vi "5_2.vi"() -> ()   [LabVIEW 2018]
uses:
  <vilib>/ptbypt/NI_PtbyPt.lvlib
  <vilib>/gmath/NI_Gmath.lvlib
panel:
  out "理论误码率":dbl
  out "噪声标准差":dbl
  out "理论门限误码率（设计误码率）":dbl
  out "理论最优门限":dbl
  out "先验概率P(H1)":dbl
  in  "先验概率P(H0)":dbl=0.5
  in  "噪声方差":dbl=0.02
  in  "样本数":u64=1000000
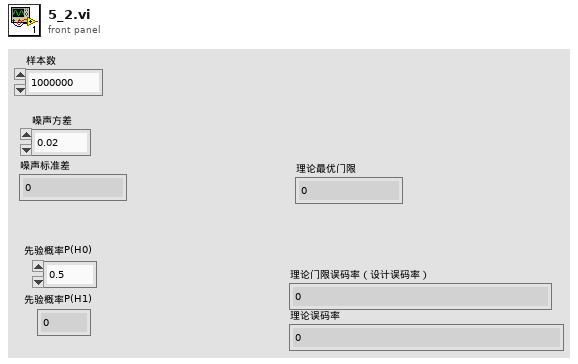
[diagram p1: front panel]
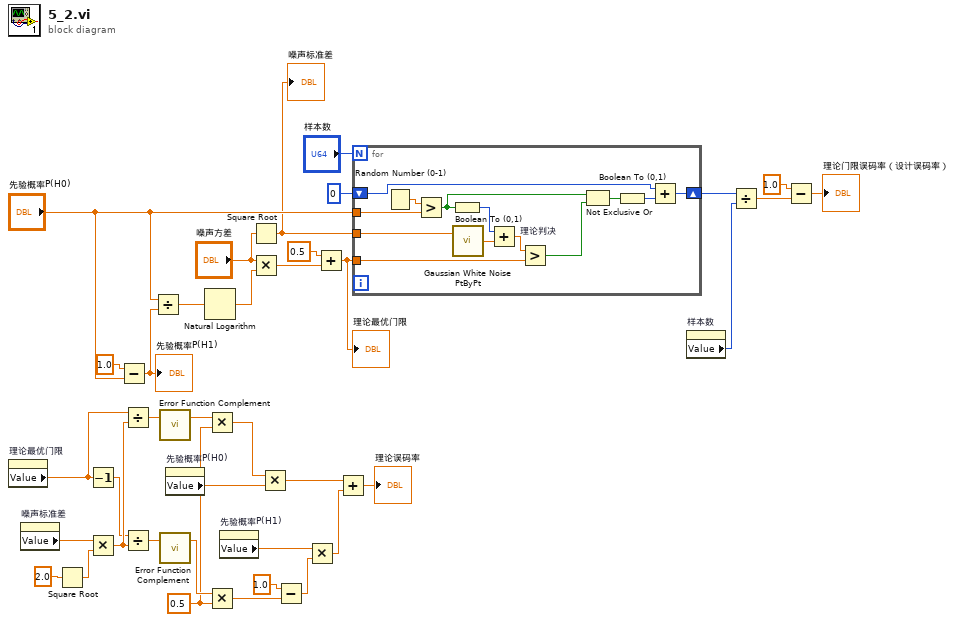
[diagram p0: block diagram]
diagram:
  w13 = 0.5 ("y")
  n1 = property on="理论最优门限" class="DigNum (严格)"() -> ("Value"=w19:dbl)  [unwired: 2 in, 2 out]
  n2 = property on="噪声标准差" class="DigNum (严格)"() -> ("Value"=w22:dbl)  [unwired: 2 in, 2 out]
  n3 = Square Root(x=2.0) -> (sqrt(x)=w21:dbl)
  n4 = Decrement(x=w19) -> (x-1=w18:dbl)
  n5 = Multiply(x=w22, y=w21) -> (x*y=w20:dbl)
  n6 = Subtract(x=1.0, y="先验概率P(H0)") -> (x-y=w29:dbl)
  "先验概率P(H1)" <- w29
  n7 = Divide(x=w19, y=w20) -> (x/y=w17:dbl)
  n8 = Divide(x=w18, y=w20) -> (x/y=w16:dbl)
  n9 = Divide(x="先验概率P(H0)", y=w29) -> (x/y=w35:dbl)
  n10 = call <vilib>:"Error Function Complement.vi"("x"=w17) -> ("1 - erf(x)"=w14:dbl)  [unwired: 2 in]
  n11 = call <vilib>:"Error Function Complement.vi"("x"=w16) -> ("1 - erf(x)"=w15:dbl)  [unwired: 2 in]
  n12 = property on="先验概率P(H0)" class="DigNum (严格)"() -> ("Value"=w5:dbl)  [unwired: 2 in, 2 out]
  n13 = Natural Logarithm(1:w35) -> (0:w34:dbl)
  n14 = Multiply(x=w14, y=w13) -> (x*y=w6:dbl)
  n15 = Multiply(x=w15, y=w13) -> (x*y=w12:dbl)
  n16 = property on="先验概率P(H1)" class="DigNum (严格)"() -> ("Value"=w4:dbl)  [unwired: 2 in, 2 out]
  n17 = Square Root(x="噪声方差") -> (sqrt(x)=w24:dbl)
  "噪声标准差" <- w24
  n18 = Multiply(x="噪声方差", y=w34) -> (x*y=w33:dbl)
  n19 = Multiply(x=w6, y=w5) -> (x*y=w1:dbl)
  n20 = Subtract(x=1.0, y=w12) -> (x-y=w3:dbl)
  n21 = Multiply(x=w4, y=w3) -> (x*y=w2:dbl)
  n22 = Add(x=0.5, y=w33) -> (x+y=w26:dbl)
  "理论最优门限" <- w26
  n23 = Add(x=w1, y=w2) -> (x+y=→"理论误码率":dbl)
  n24 = for {
    N: "样本数" -> [_]
    tunnel: w24 -> [w50]
    tunnel: "先验概率P(H0)" -> [w47]
    tunnel: w26 -> [w46]
    shift-right: [w44] -> w25
    shift-left: u64 0 ("元素") -> [w42]
    n25 = Random Number (0-1)() -> (number: 0 to 1=w48:dbl)
    n26 = Greater?(x=w48, y=w47) -> (0:w38:bool)
    n27 = Boolean To (0,1)(Boolean=w38) -> (0, 1=w41:i16)
    n28 = call <vilib>:"Gaussian White Noise PtByPt.vi"("standard deviation"=w50) -> ("Gaussian white noise"=w49:dbl)  [unwired: 2 in]
    n29 = Add(x=w41, y=w49) -> (x+y=w39:dbl)
    n30 = Greater? "理论判决"(x=w39, y=w46) -> (0:w45:bool)
    n31 = Not Exclusive Or(1:w45, 2:w38) -> (0:w40:bool)
    n32 = Boolean To (0,1)(Boolean=w40) -> (0, 1=w43:i16)
    n33 = Add(x=w42, y=w43) -> (x+y=w44:u64)
  }
  n34 = property on="样本数" class="DigNum (严格)"() -> ("Value"=w27:u64)  [unwired: 2 in, 2 out]
  n35 = Divide(x=w25, y=w27) -> (x/y=w9:dbl)
  n36 = Subtract(x=1.0, y=w9) -> (x-y=→"理论门限误码率（设计误码率）":dbl)
